vi "Camera Manager Load Param.vi"(8 "error in (no error)":errorcluster, 11 "cameraId":i32) -> (0 "error out":errorcluster)   [LabVIEW 2017, in "PlayNitrideCameraComponet1010_4.lvlib"]
doc: "__declspec(dllexport) void CameraManager_LoadParam(int cameraId);"
uses:
  <userlib>/PlayNitrideCameraComponet1010_4/PlayNitrideCameraComponet1010_4.lvlib
  <userlib>/PlayNitrideCameraComponet1010_4/PlayNitrideCameraComponet.dll
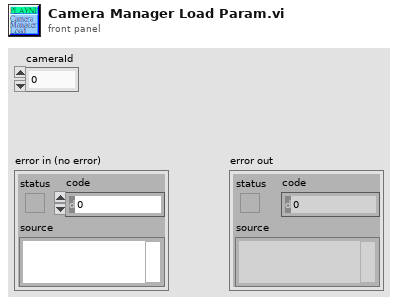
[diagram p1: front panel]
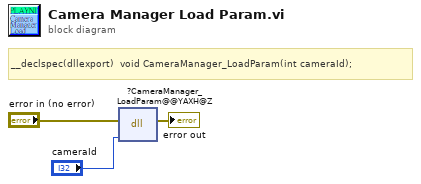
[diagram p0: block diagram]
diagram:
  # "__declspec(dllexport)  void CameraManager_LoadParam(int cameraId);"
  n1 = dll-call lib="C:/Program Files/National Instruments/LabVIEW 2017/user.lib/PlayNitrideCameraComponet1010_4/PlayNitrideCameraComponet.*" fn="?CameraManager_LoadParam@@YAXH@Z"(error in="error in (no error)", "cameraId"="cameraId") -> (error out=→"error out":errorcluster)  [unwired: 4 in, 1 out]
